vi "Write to File.vi"(8 "Error In":errorcluster, 11 "APDClass.lvclass":refnum<class "APDClass.lvclass">) -> (0 "Error Out":errorcluster)   [LabVIEW 2020, in "APDClass.lvclass"]
uses:
  APDClass.lvclass
  APDClass.lvclass/APDClass.ctl
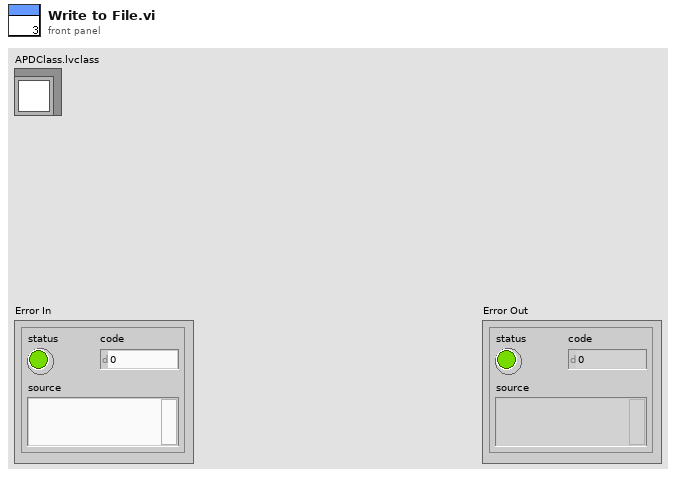
[diagram p1: front panel]
types:
  T1 = enum16{"open", "open or create", "create or replace", "create", "open (read-only)"}
  T2 = typedef "GainData.ctl" = cluster{"CtrlV":dbl[], "NumOfWFs":i32, "WF length":i32, "Gain":dbl[], "GainRaw":dbl[][], "GainBGRaw":dbl[][]}
  T3 = typedef "iRFData.ctl" = cluster{"dt":dbl, "NumOfWFs":i32, "WFLength":i32, "iRFCtrlV":dbl[], "iRFWFsAvg":dbl[][], "iRFRaw":dbl[][]}
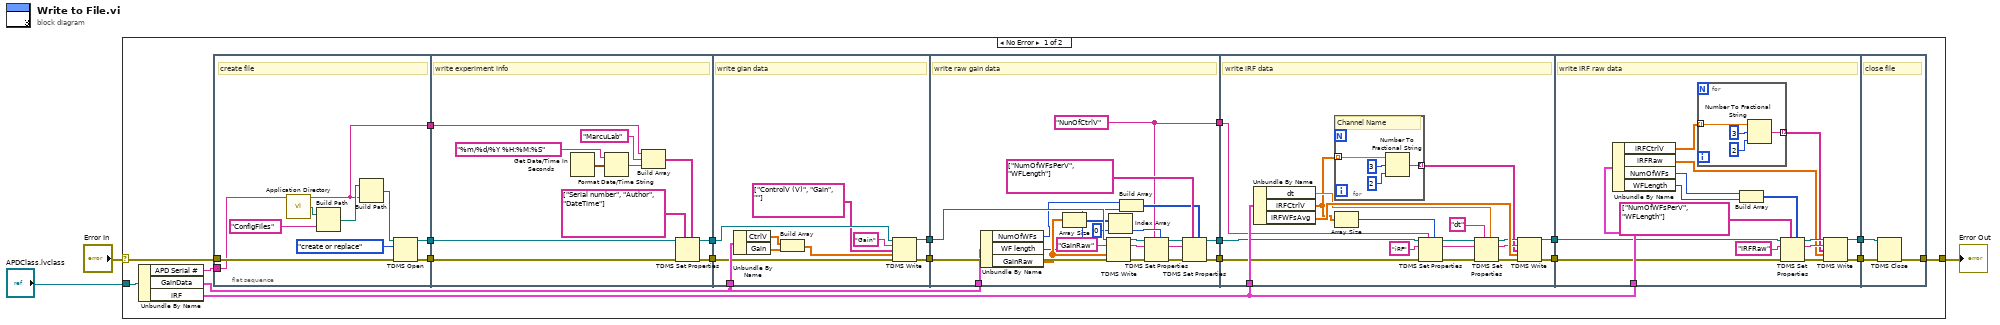
[diagram p0: block diagram]
diagram:
  n1 = case shown="No Error" "Error In" {
    selector: "Error In" -> [w22 w121]
    tunnel: [w13 w121] -> w2
    tunnel: "APDClass.lvclass" -> [w23 _]
    frame No Error {
      n2 = Unbundle By Name(w23) -> ("APD Serial #"=w19:string, "GainData"=w6:T2, "iRF"=w5:T3)
      n3 = flat-sequence {
        tunnel: w22 -> [w29]
        tunnel: w19 -> [w24]
        tunnel: [w26] -> w21
        tunnel: [w25] -> w20
        tunnel: [w24] -> w18
        tunnel: w21 -> [w38]
        tunnel: w20 -> [w37]
        tunnel: w18 -> [w33]
        tunnel: [w36] -> w17
        tunnel: [w35] -> w16
        tunnel: w17 -> [w50]
        tunnel: w16 -> [w52]
        tunnel: w6 -> [w53]
        tunnel: [w46] -> w8
        tunnel: [w45] -> w7
        tunnel: [w64] -> w10
        tunnel: [w63] -> w9
        tunnel: w8 -> [w74]
        tunnel: w7 -> [w72]
        tunnel: w6 -> [w68]
        tunnel: [w54] -> w4
        tunnel: w10 -> [w84]
        tunnel: w9 -> [w82]
        tunnel: w5 -> [w93]
        tunnel: [w78] -> w15
        tunnel: [w77] -> w14
        tunnel: w4 -> [w85]
        tunnel: w15 -> [w104]
        tunnel: w14 -> [w106]
        tunnel: w5 -> [w113]
        tunnel: [w103] -> w12
        tunnel: [w102] -> w11
        tunnel: [w120] -> w13
        tunnel: w12 -> [w119]
        tunnel: w11 -> [w118]
        frame #0 {
          # "create file"
          n4 = call <vilib>:"Application Directory.vi"() -> ("Application Directory"=w30:path)
          n5 = Build Path(base path=w30, name or relative path="ConfigFiles") -> (appended path=w31:path)
          n6 = Build Path(base path=w31, name or relative path=w24) -> (appended path=w32:path)
          n7 = TDMS Open(8:w29, 10:T1."create or replace" ("operation (0:open)"), 11:w32) -> (0:w26:errorcluster, 3:w25:refnum<k34>)  [unwired: 4 in]
        }
        frame #1 {
          # "write experiment info"
          n8 = Get Date/Time In Seconds() -> (seconds since 1Jan1904=w42:timestamp)
          n9 = Format Date/Time String(time format string (%c)="%m/%d/%Y %H:%M:%S", seconds (now)=w42) -> (date/time string=w43:string)  [unwired: 1 in]
          n10 = Build Array(w33, "MarcuLab" ("element"), w43) -> (w34:string[])
          n11 = TDMS Set Properties(5:w34, 7:string[] ["Serial number", "Author", "DateTime"] ("property names"), 8:w38, 11:w37) -> (0:w36:errorcluster, 3:w35:refnum<k34>)  [unwired: 2 in, 2 out]
        }
        frame #2 {
          # "write gian data"
          n12 = Unbundle By Name(w53) -> ("CtrlV"=w44:dbl[], "Gain"=w49:dbl[])
          n13 = Build Array(w44, w49) -> (w48:dbl[][])
          n14 = TDMS Write(0:w52, 5:"Gain" ("group name in (Untitled)"), 7:string[] ["ControlV (V)", "Gain", ""] ("channel name(s) in (Untitled)"), 9:w48, 11:w50) -> (4:w46:refnum<k34>, 15:w45:errorcluster)  [unwired: 1 in, 2 out]
        }
        frame #3 {
          w54 = "NunOfCtrlV"
          # "write raw gain data"
          n15 = Unbundle By Name(w68) -> ("NumOfWFs"=w60:i32, "WF length"=w59:i32, "GainRaw"=w67:dbl[][])
          n16 = Array Size(array=w67) -> (size(s)=w57:i32[])
          n17 = TDMS Write(0:w74, 5:"GainRaw" ("group name in (Untitled)"), 9:w67, 11:w72) -> (4:w71:refnum<k34>, 6:w70:string, 15:w69:errorcluster)  [unwired: 2 in, 1 out]
          n18 = Index Array(array=w57, index=0) -> (element=w55:i32)
          n19 = Build Array(w60, w59) -> (w58:i32[])
          n20 = TDMS Set Properties(5:w55, 7:w54, 8:w69, 10:w70, 11:w71) -> (0:w65:errorcluster, 2:w62:string, 3:w66:refnum<k34>)  [unwired: 1 in, 1 out]
          n21 = TDMS Set Properties(5:w58, 7:string[] ["NumOfWFsPerV", "WFLength"] ("property names"), 8:w65, 10:w62, 11:w66) -> (0:w64:errorcluster, 3:w63:refnum<k34>)  [unwired: 1 in, 2 out]
        }
        frame #4 {
          # "write iRF data"
          n22 = Unbundle By Name(w93) -> ("dt"=w80:dbl, "iRFCtrlV"=w76:dbl[], "iRFWFsAvg"=w92:dbl[][])
          n23 = for {
            tunnel: w76 -> [w95] mode=indexing
            tunnel: [w94] -> w81 mode=indexing
            # "Channel Name"
            n24 = Number To Fractional String(number=w95, width (-)=i16 3, precision (6)=i16 2) -> (F-format string=w94:string)  [unwired: 1 in]
          }
          n25 = Array Size(array=w76) -> (size(s)=w75:i32)
          n26 = TDMS Set Properties(5:w75, 7:w85, 8:w84, 10:"iRF" ("group name"), 11:w82) -> (0:w86:errorcluster, 2:w89:string, 3:w87:refnum<k34>)  [unwired: 1 in, 1 out]
          n27 = TDMS Set Properties(5:w80, 7:"dt" ("property names"), 8:w86, 10:w89, 11:w87) -> (0:w90:errorcluster, 2:w91:string, 3:w88:refnum<k34>)  [unwired: 1 in, 1 out]
          n28 = TDMS Write(0:w88, 5:w91, 7:w81, 9:w92, 11:w90) -> (4:w78:refnum<k34>, 15:w77:errorcluster)  [unwired: 1 in, 2 out]
        }
        frame #5 {
          # "write iRF raw data"
          n29 = Unbundle By Name(w113) -> ("iRFCtrlV"=w101:dbl[], "iRFRaw"=w108:dbl[][], "NumOfWFs"=w100:i32, "WFLength"=w99:i32)
          n30 = for {
            tunnel: [w117] -> w109 mode=indexing
            tunnel: w101 -> [w116] mode=indexing
            n31 = Number To Fractional String(number=w116, width (-)=i16 3, precision (6)=i16 2) -> (F-format string=w117:string)  [unwired: 1 in]
          }
          n32 = Build Array(w100, w99) -> (w98:i32[])
          n33 = TDMS Set Properties(5:w98, 7:string[] ["NumOfWFsPerV", "WFLength"] ("property names"), 8:w106, 10:"iRFRaw" ("group name"), 11:w104) -> (0:w111:errorcluster, 2:w112:string, 3:w110:refnum<k34>)  [unwired: 1 in, 1 out]
          n34 = TDMS Write(0:w110, 5:w112, 7:w109, 9:w108, 11:w111) -> (4:w103:refnum<k34>, 15:w102:errorcluster)  [unwired: 1 in, 2 out]
        }
        frame #6 {
          # "close file"
          n35 = TDMS Close(8:w118, 11:w119) -> (0:w120:errorcluster)  [unwired: 1 out]
        }
      }
    }
    frame Error {
    }
  }
  "Error Out" <- w2
